vi "总磷总氮通讯.vi"() -> ()   [LabVIEW 2016, in "斯坦道仪器.lvlib"]
uses:
  <vilib>/Utility/config.llb/Write Key (Boolean).vi
  <vilib>/Utility/config.llb/Write Key (String).vi
  <vilib>/Utility/config.llb/Read Key (Boolean).vi
  <vilib>/Utility/config.llb/Read Key (String).vi
  <vilib>/Plasmionique/MB Master/MB_Master/MB_Master.lvclass
  <vilib>/Utility/config.llb/NI_LVConfig.lvlib
  <vilib>/Plasmionique/MB Master/MB Master.lvlib
  <vilib>/ptbypt/NI_PtbyPt.lvlib
panel:
  out "序列号":string
  out "状态告警区":T1
  out "测量数据区":T2 {"单位" items=["ug/L", "mg/L", "ppm", "mg/m3", "cm", "ppb", "ug/m3", "%", "nmol/mol", "umol/mol", "MPN/L", "MPN/100ml", "ng/m3", "NTU", "无量纲", "ms/cm", "us/cm", "℃", "mV", "万个/L"]}
  out "status":bool
  out "关键参数区":T3
  in  "读关键参数区":bool
  in  "读状态告警区":bool
  in  "读测量数据区":bool
  in  "站号":u16(ring) items=["总磷"=1, "氨氮"=3]
  in  "停止":bool
  in  "启动":bool
  in  "控制命令":u16(ring) items=["启动测量"=1, "标样核查"=2, "零点核查"=3, "跨度核查"=4, "空白测试"=5, "平行样测试"=6, "加标回收"=7, "空白校准"=8, "标样校准"=9, "初始化（清洗）"=10, "停止测试"=11, "仪器重启"=12, "校时"=13, "模式设置"=14, "测量间隔设置"=15]
  in  "控制命令参数":u16[](array[numeric]) format="%04xH"
  in  "VISA Resource":refnum<visa-resource-name>
  in  "启用模块":bool
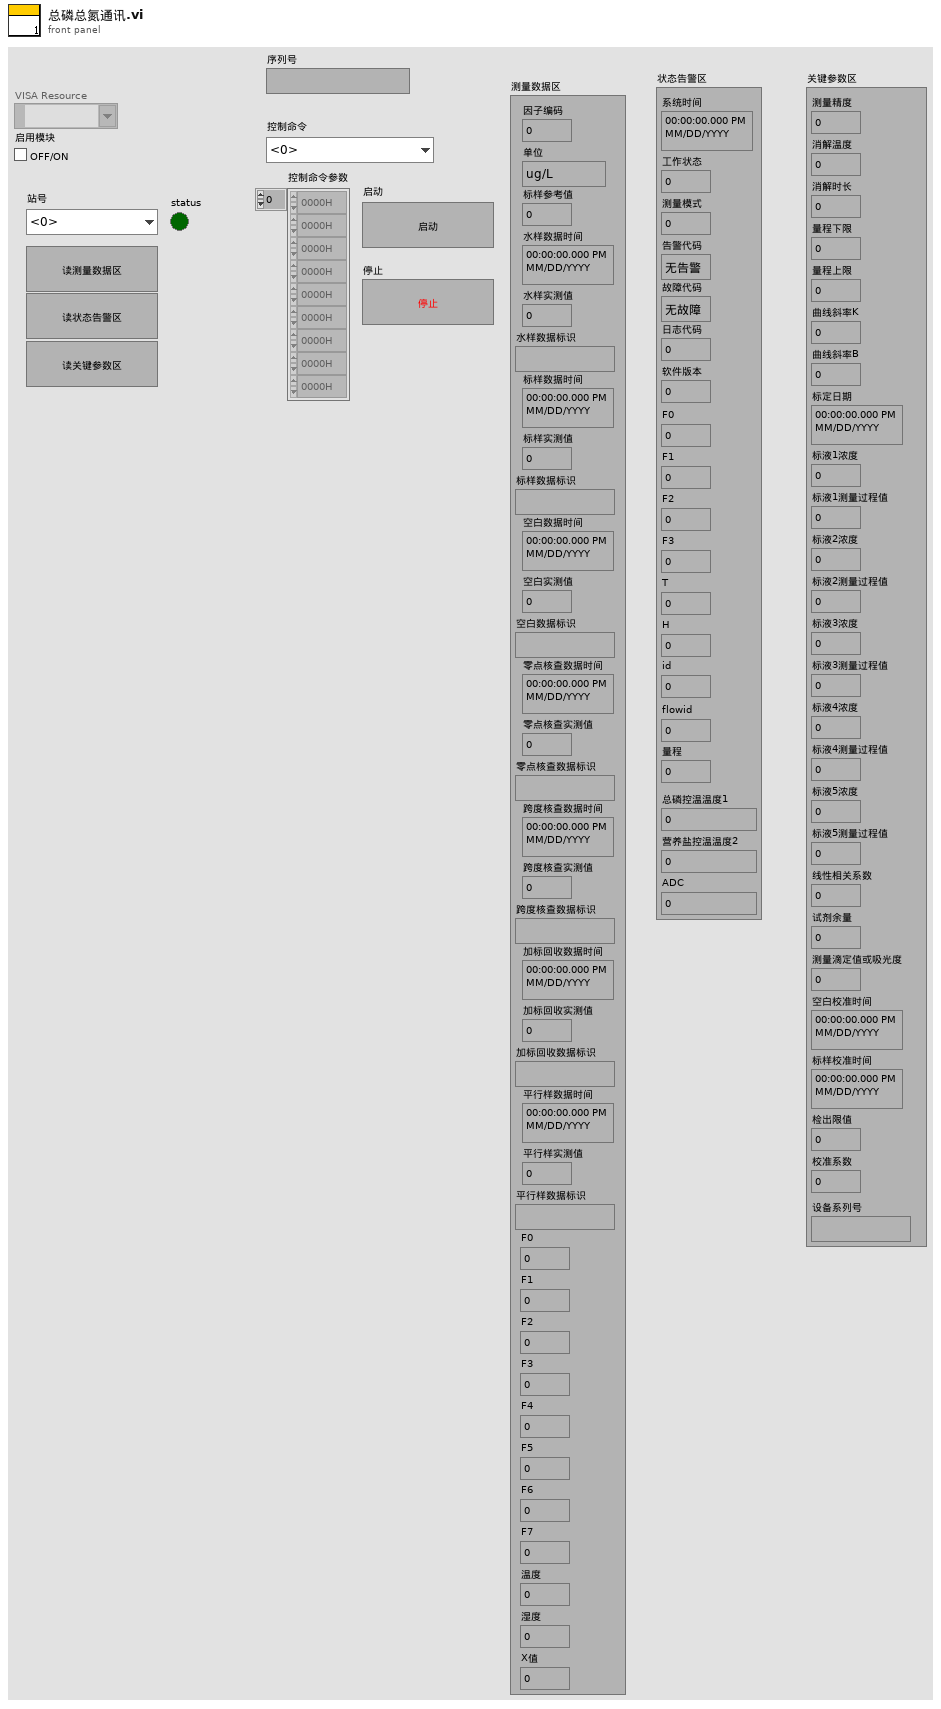
[diagram p1: front panel]
types:
  T1 = cluster{"系统时间":timestamp, "工作状态":u16, "测量模式":u16, "告警代码":enum16{"无告警", "缺试剂告警", "缺水样告警", "缺蒸馏水告警", "缺标液告警", "仪表漏液告警", "标定异常告警", "超量程告警", "加热异常", "低试剂预警", "超上限告警", "超下限告警", "仪表内部其他异常", "滴定异常告警", "电极异常告警", "量程切换告警", "参数设置告警", "PH电极电位异常", "电导率电极异常", "浊度光度异常", "溶解氧电极异常", "溶解氧光强异常", "温度异常告警", "PH异常告警", "溶解氧异常告警", "电导率异常告警", "浊度异常告警", "叶绿素异常告警", "藻密度异常告警", "蓝绿藻异常告警", "ORP异常告警", "氨氮异常告警", "清洁刷异常告警", "SD卡异常告警", "蓝牙异常告警", "Wifi异常告警", "流程异常告警"}, "故障代码":enum16{"无故障", "电机故障", "温度故障", "通讯故障", "滴定故障"}, "日志代码":u16, "软件版本":u16, "F0":sgl, "F1":sgl, "F2":sgl, "F3":sgl, "T":sgl, "H":sgl, "id":u16, "flowid":u16, "量程":u16, "总磷控温温度1":sgl, "营养盐控温温度2":sgl, "ADC":sgl}
  T2 = cluster{"因子编码":u32, "单位":u16, "标样参考值":sgl, "水样数据时间":timestamp, "水样实测值":sgl, "水样数据标识":string, "标样数据时间":timestamp, "标样实测值":sgl, "标样数据标识":string, "空白数据时间":timestamp, "空白实测值":sgl, "空白数据标识":string, "零点核查数据时间":timestamp, "零点核查实测值":sgl, "零点核查数据标识":string, "跨度核查数据时间":timestamp, "跨度核查实测值":sgl, "跨度核查数据标识":string, "加标回收数据时间":timestamp, "加标回收实测值":sgl, "加标回收数据标识":string, "平行样数据时间":timestamp, "平行样实测值":sgl, "平行样数据标识":string, "F0":sgl, "F1":sgl, "F2":sgl, "F3":sgl, "F4":sgl, "F5":sgl, "F6":sgl, "F7":sgl, "温度":sgl, "湿度":sgl, "X值":sgl}
  T3 = cluster{"测量精度":u16, "消解温度":u16, "消解时长":u16, "量程下限":sgl, "量程上限":sgl, "曲线斜率K":sgl, "曲线斜率B":sgl, "标定日期":timestamp, "标液1浓度":sgl, "标液1测量过程值":sgl, "标液2浓度":sgl, "标液2测量过程值":sgl, "标液3浓度":sgl, "标液3测量过程值":sgl, "标液4浓度":sgl, "标液4测量过程值":sgl, "标液5浓度":sgl, "标液5测量过程值":sgl, "线性相关系数":sgl, "试剂余量":u32, "测量滴定值或吸光度":sgl, "空白校准时间":timestamp, "标样校准时间":timestamp, "检出限值":sgl, "校准系数":sgl, "设备系列号":string}
  T4 = typedef "NI_LVConfig.lvlib/Config Data RefNum.ctl" = refnum<k1>
  T5 = enum8{"Enabled", "Disabled", "Disabled and Grayed Out"}
  T6 = cluster{"系统时间":timestamp, "工作状态":enum16{"空闲", "水样测试", "标样核查", "零点核查", "跨度核查", "空白测试", "平行样测试", "加标回收", "空白校准", "标样校准", "初始化（清洗）"}, "测量模式":enum16{"待机", "连续模式", "周期模式", "定点模式", "受控模式", "手动模式"}, "告警代码":enum16{"无告警", "缺试剂告警", "缺水样告警", "缺蒸馏水告警", "缺标液告警", "仪表漏液告警", "标定异常告警", "超量程告警", "加热异常", "低试剂预警", "超上限告警", "超下限告警", "仪表内部其他异常", "滴定异常告警", "电极异常告警", "量程切换告警", "参数设置告警", "PH电极电位异常", "电导率电极异常", "浊度光度异常", "溶解氧电极异常", "溶解氧光强异常", "温度异常告警", "PH异常告警", "溶解氧异常告警", "电导率异常告警", "浊度异常告警", "叶绿素异常告警", "藻密度异常告警", "蓝绿藻异常告警", "ORP异常告警", "氨氮异常告警", "清洁刷异常告警", "SD卡异常告警", "蓝牙异常告警", "Wifi异常告警", "流程异常告警"}, "故障代码":enum16{"无故障", "电机故障", "温度故障", "通讯故障", "滴定故障"}, "日志代码":u16, "软件版本":u16, "F0":sgl, "F1":sgl, "F2":sgl, "F3":sgl, "T":sgl, "H":sgl, "id":u16, "flowid":u16, "量程":u16, "总磷控温温度1":sgl, "营养盐控温温度2":sgl, "ADC":sgl}
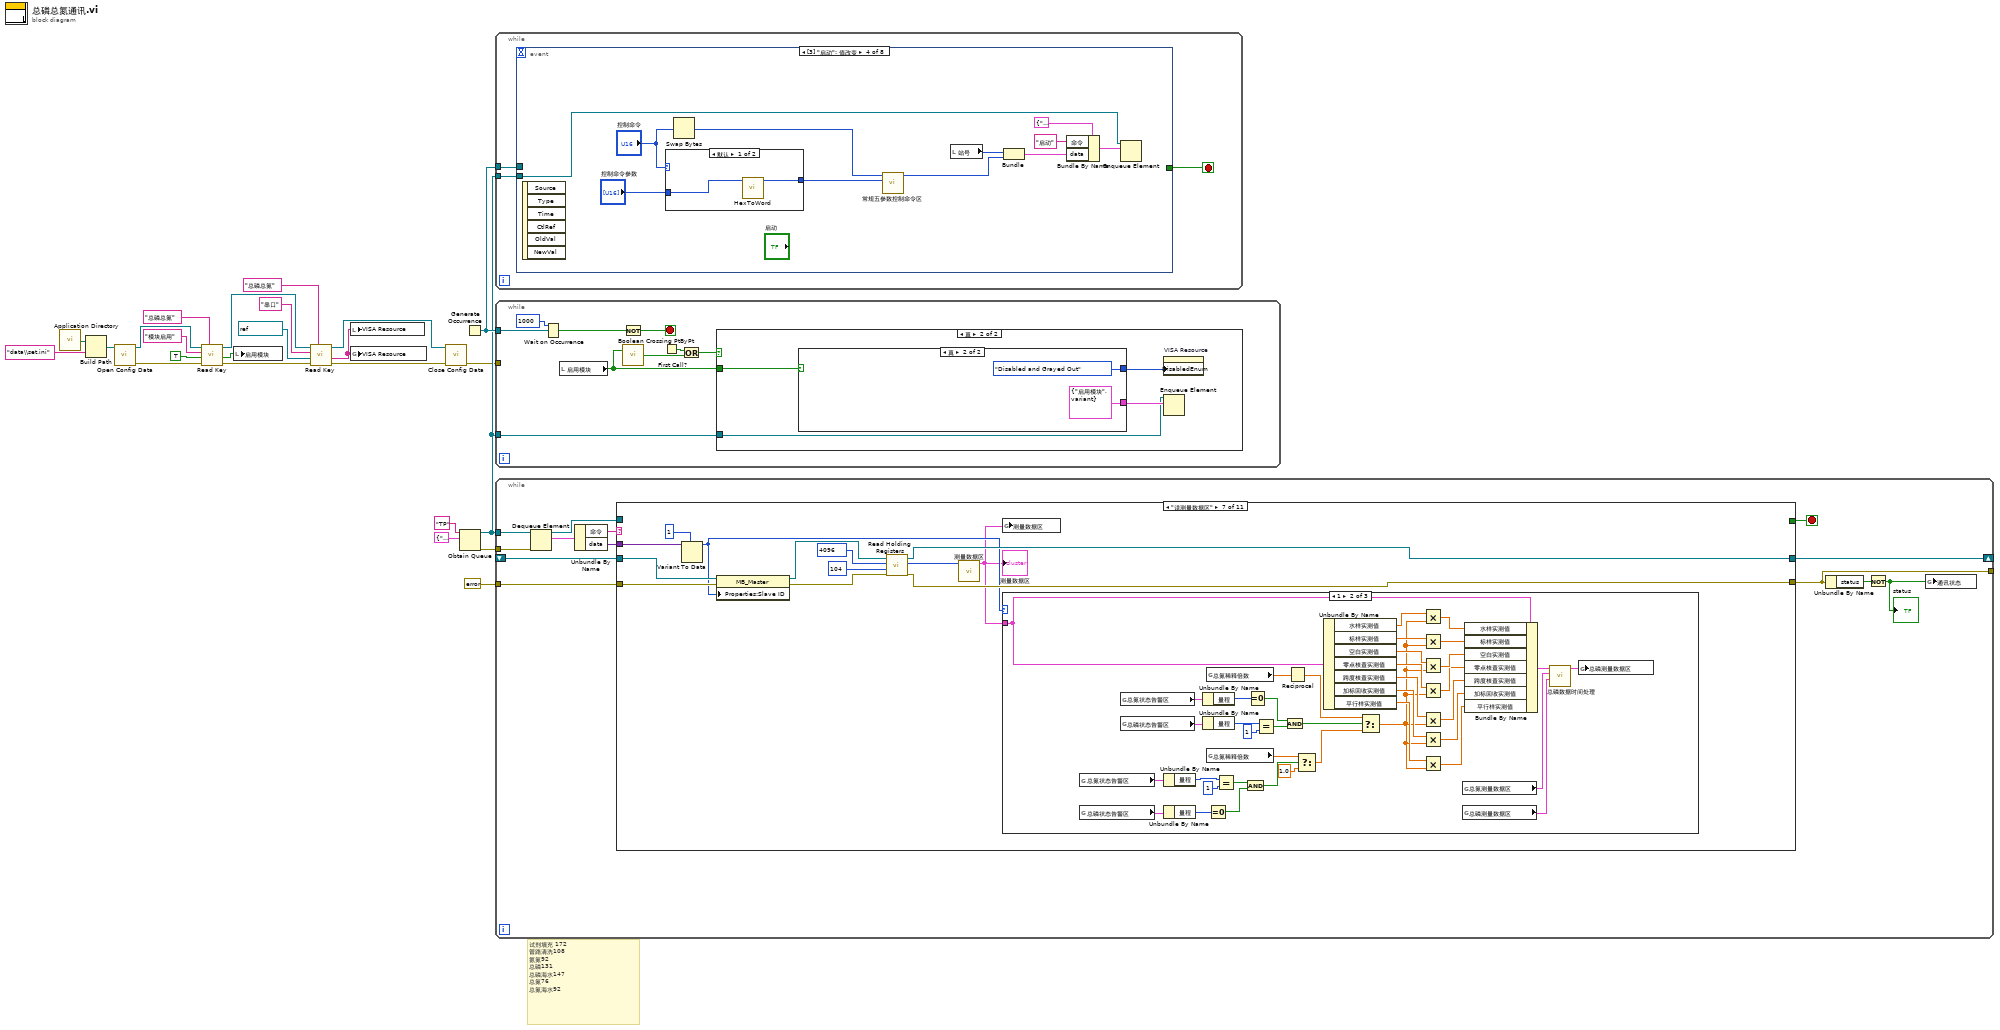
[diagram p0: block diagram]
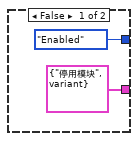
[diagram p3: hidden frame]
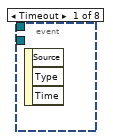
[diagram p4: hidden frame]
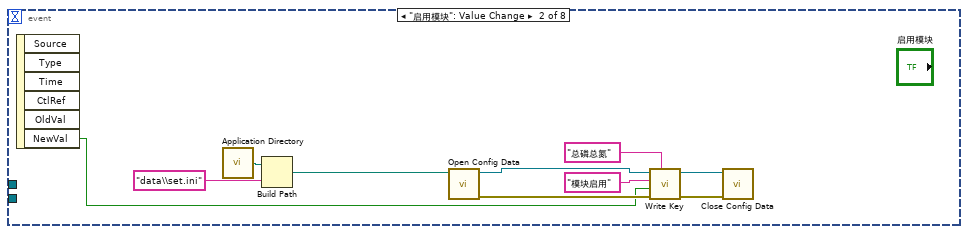
[diagram p5: hidden frame]
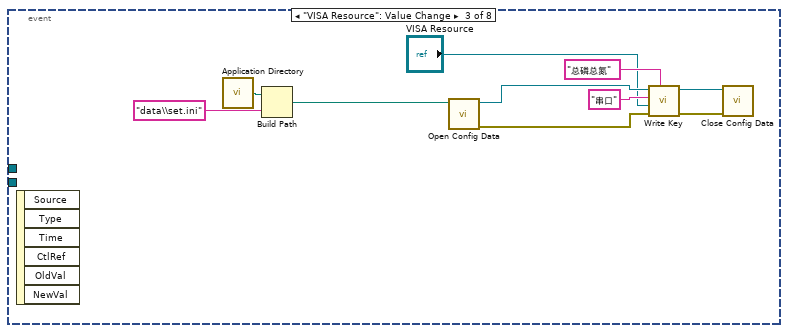
[diagram p6: hidden frame]
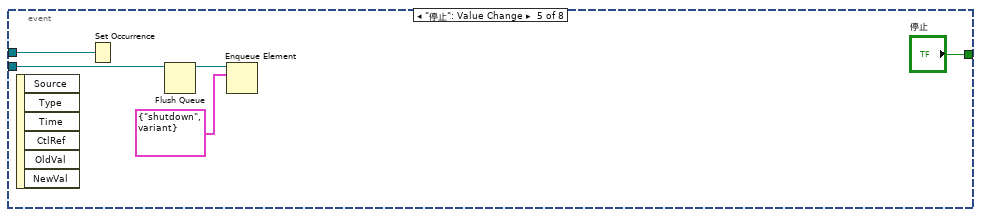
[diagram p8: hidden frame]
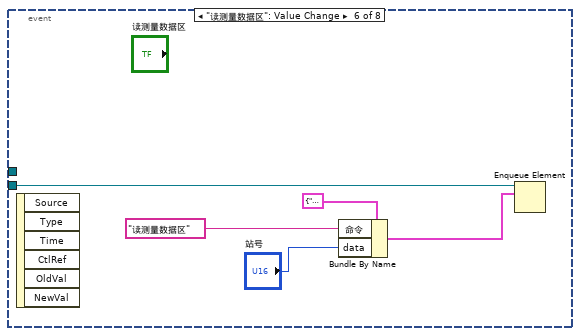
[diagram p9: hidden frame]
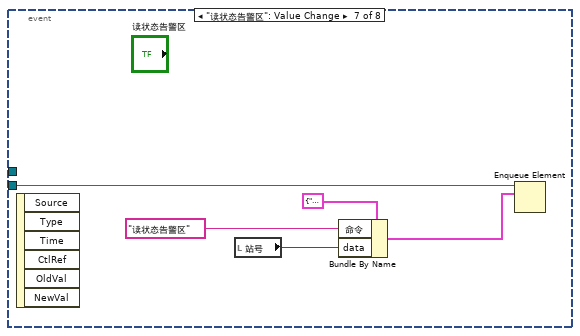
[diagram p10: hidden frame]
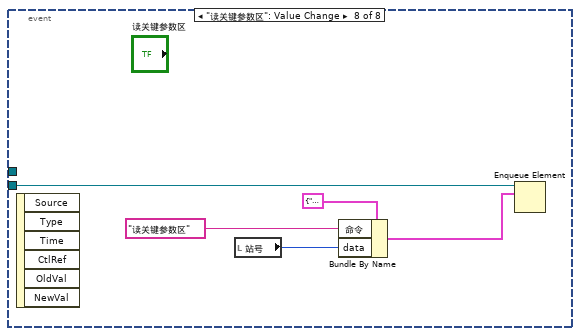
[diagram p11: hidden frame]
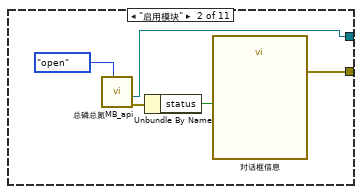
[diagram p13: hidden frame]
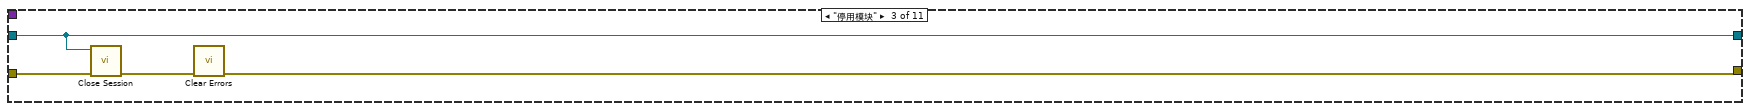
[diagram p14: hidden frame]
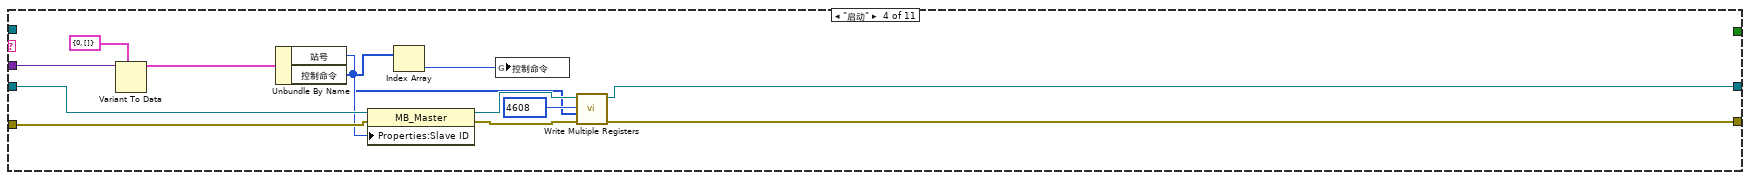
[diagram p15: hidden frame]
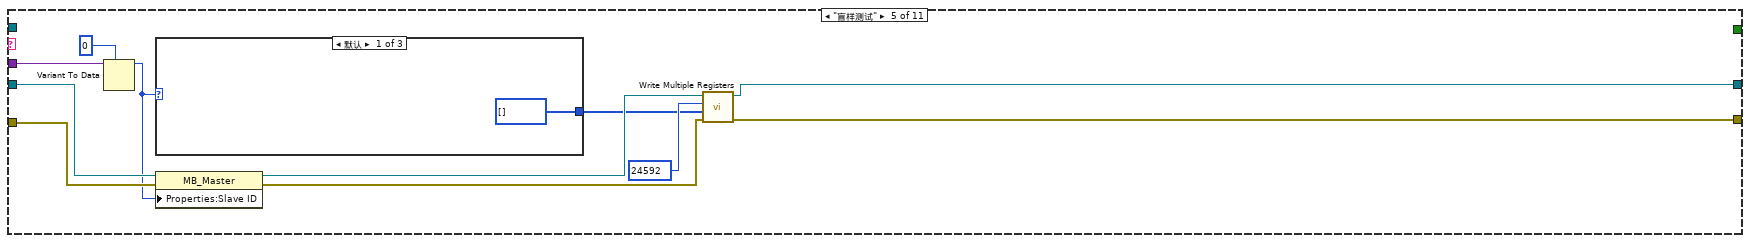
[diagram p16: hidden frame]
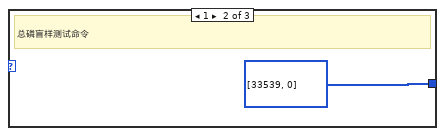
[diagram p17: hidden frame]
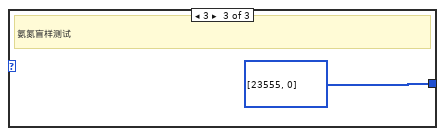
[diagram p18: hidden frame]
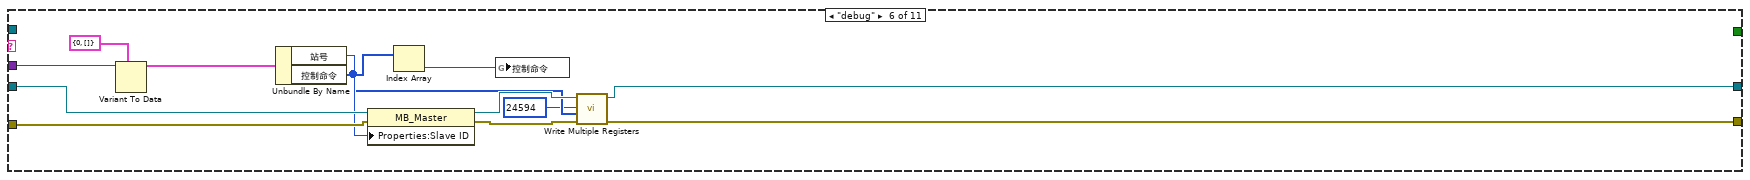
[diagram p19: hidden frame]
diagram:
  # "试剂填充 172 \n管路清洗108\n氨氮92\n总磷131\n总磷海水147\n总氮76\n总氮海水92"
  n1 = call <vilib>:"Application Directory.vi"() -> ("Application Directory"=w12:path)
  n2 = Build Path(base path=w12, name or relative path="data\\set.ini" ("名称或相对路径")) -> (appended path=w13:path)
  n3 = call <vilib>:"Open Config Data.vi"("configuration file path"=w13) -> ("error out"=w18:errorcluster, "refnum"=w17:T4)  [unwired: 8 in, 1 out]
  n4 = call-poly <vilib>:"Read Key.vi"("section"="总磷总氮", "error in (no error)"=w18, "default value"=TRUE ("启用模块"), "key"="模块启用", "refnum"=w17) -> ("error out"=w6:errorcluster, "value"=w9:bool, "refnum out"=w8:T4)  [unwired: 3 in, 1 out]
  n5 = local write "启用模块"(w9) -> ()
  n6 = call-poly <vilib>:"Read Key.vi"("section"="总磷总氮", "error in (no error)"=w6, "default value"=refnum<visa-resource-name> "COM5" ("VISA Resource"), "key"="串口", "refnum"=w8) -> ("error out"=w5:errorcluster, "value"=w1:string, "refnum out"=w7:T4)  [unwired: 3 in, 1 out]
  n7 = local write "VISA Resource"(w1) -> ()
  n8 = global write "VAR总磷总氮全局变量.vi" "VISA Resource"(w1) -> ()
  n9 = call <vilib>:"Close Config Data.vi"("error in (no error)"=w5, "refnum"=w7) -> ("error out"=w10:errorcluster)  [unwired: 8 in, 1 out]
  n10 = Obtain Queue(name (unnamed)="TP" ("名称（未命名）"), element data type=cluster{"命令":string, "data":variant} {"命令"="", "data"=variant}) -> (queue out=w19:refnum<queue>, error out=w22:errorcluster)  [unwired: 3 in, 1 out]
  n11 = Generate Occurrence() -> (w20:refnum<k4>)
  n12 = while {
    tunnel: w19 -> [w27]
    tunnel: w20 -> [w25]
    stop <- w26 stop-if-true
    n13 = event shown="[3] \"启动\": 值改变" {
      selector: _ -> [_ _ _ _ _ _ _ _]
      dyn-events: _ -> [_ _ _ _ _ _ _ _]
      timeout: _ -> [_ _ _ _ _ _ _ _]
      tunnel: w27 -> [_ _ _ w58 w65 w71 w76 w81]
      tunnel: [_ _ _ _ "停止" _ _ _] -> w26
      tunnel: w25 -> [_ _ _ _ w62 _ _ _]
      event Timeout {
        n14 = event-data() -> ()  [unwired: 1 in, 3 out]
      }
      event "启用模块": Value Change {
        n15 = event-data() -> ("NewVal"=w28:bool)  [unwired: 1 in, 5 out]
        n16 = call <vilib>:"Application Directory.vi"() -> ("Application Directory"=w30:path)
        n17 = Build Path(base path=w30, name or relative path="data\\set.ini" ("名称或相对路径")) -> (appended path=w31:path)
        n18 = call <vilib>:"Open Config Data.vi"("configuration file path"=w31) -> ("error out"=w37:errorcluster, "refnum"=w36:T4)  [unwired: 8 in, 1 out]
        n19 = call-poly <vilib>:"Write Key.vi"("section"="总磷总氮", "error in (no error)"=w37, "value"=w28, "key"="模块启用", "refnum"=w36) -> ("error out"=w33:errorcluster, "refnum out"=w29:T4)  [unwired: 4 in, 1 out]
        n20 = call <vilib>:"Close Config Data.vi"("error in (no error)"=w33, "refnum"=w29) -> ()  [unwired: 8 in, 2 out]
      }
      event "VISA Resource": Value Change {
        n21 = event-data() -> ()  [unwired: 1 in, 6 out]
        n22 = call <vilib>:"Application Directory.vi"() -> ("Application Directory"=w40:path)
        n23 = Build Path(base path=w40, name or relative path="data\\set.ini" ("名称或相对路径")) -> (appended path=w41:path)
        n24 = call <vilib>:"Open Config Data.vi"("configuration file path"=w41) -> ("error out"=w47:errorcluster, "refnum"=w46:T4)  [unwired: 8 in, 1 out]
        n25 = call-poly <vilib>:"Write Key.vi"("section"="总磷总氮", "error in (no error)"=w47, "value"="VISA Resource", "key"="串口", "refnum"=w46) -> ("error out"=w43:errorcluster, "refnum out"=w39:T4)  [unwired: 4 in, 1 out]
        n26 = call <vilib>:"Close Config Data.vi"("error in (no error)"=w43, "refnum"=w39) -> ()  [unwired: 8 in, 2 out]
      }
      event "启动": Value Change {
        n27 = event-data() -> ()  [unwired: 1 in, 6 out]
        n28 = case shown="默认" "控制命令" {
          tunnel: "控制命令参数" -> [w60 w61]
          tunnel: [w59 w61] -> w48
          frame Default {
            n29 = call "HexToWord.vi"("数组"=w60) -> ("WORD"=w59:u16[])  [unwired: 10 in]
          }
          frame 13 {
          }
        }
        n30 = Swap Bytes(anything="控制命令") -> (byte swapped=w51:u16)
        n31 = call "常规五参数控制命令区.vi"("控制命令参数"=w48, "控制命令"=w51) -> ("控制命令输出"=w54:u16[])  [unwired: 9 in]
        n32 = local read "站号"() -> (w53:u16)
        n33 = Bundle("站号"=w53, "控制命令输出"=w54) -> (w52:cluster{"站号":u16, "控制命令输出":u16[]})  [unwired: 1 in]
        n34 = Bundle By Name(cluster=cluster{"命令":string, "data":variant} {"命令"="", "data"=variant} ("元素"), "命令"="启动", "data"=w52) -> (w56:cluster{"命令":string, "data":variant})
        n35 = Enqueue Element(queue=w58, element=w56) -> ()  [unwired: 2 in, 3 out]
      }
      event "停止": Value Change {
        n36 = event-data() -> ()  [unwired: 1 in, 6 out]
        n37 = Set Occurrence(w62) -> ()
        n38 = Flush Queue(queue=w65) -> (queue out=w64:refnum<queue>)  [unwired: 1 in, 2 out]
        n39 = Enqueue Element(queue=w64, element=cluster{"命令":string, "data":variant} {"命令"="shutdown", "data"=variant} ("元素")) -> ()  [unwired: 2 in, 3 out]
      }
      event "读测量数据区": Value Change {
        n40 = event-data() -> ()  [unwired: 1 in, 6 out]
        n41 = Bundle By Name(cluster=cluster{"命令":string, "data":variant} {"命令"="", "data"=variant} ("元素"), "命令"="读测量数据区", "data"="站号") -> (w69:cluster{"命令":string, "data":variant})
        n42 = Enqueue Element(queue=w71, element=w69) -> ()  [unwired: 2 in, 3 out]
      }
      event "读状态告警区": Value Change {
        n43 = event-data() -> ()  [unwired: 1 in, 6 out]
        n44 = local read "站号"() -> (w72:u16)
        n45 = Bundle By Name(cluster=cluster{"命令":string, "data":variant} {"命令"="", "data"=variant} ("元素"), "命令"="读状态告警区", "data"=w72) -> (w74:cluster{"命令":string, "data":variant})
        n46 = Enqueue Element(queue=w76, element=w74) -> ()  [unwired: 2 in, 3 out]
      }
      event "读关键参数区": Value Change {
        n47 = event-data() -> ()  [unwired: 1 in, 6 out]
        n48 = local read "站号"() -> (w77:u16)
        n49 = Bundle By Name(cluster=cluster{"命令":string, "data":variant} {"命令"="", "data"=variant} ("元素"), "命令"="读关键参数区", "data"=w77) -> (w79:cluster{"命令":string, "data":variant})
        n50 = Enqueue Element(queue=w81, element=w79) -> ()  [unwired: 2 in, 3 out]
      }
    }
  }
  n51 = while {
    tunnel: w20 -> [w90]
    tunnel: w19 -> [w85]
    tunnel: w10 -> [_]
    stop <- w87 stop-if-true
    n52 = Wait on Occurrence(2:w90, 3:1000 ("毫秒超时(-1)")) -> (0:w88:bool)  [unwired: 1 in]
    n53 = local read "启用模块"() -> (w86:bool)
    n54 = Not(x=w88) -> (.not. x?=w87:bool)
    n55 = call <vilib>:"Boolean Crossing PtByPt.vi"("input"=w86) -> ("crossing"=w83:bool)  [unwired: 2 in]
    n56 = First Call?() -> (First Call?: T/F=w84:bool)
    n57 = Or(x=w84, y=w83) -> (x .or. y?=w82:bool)
    n58 = case shown="真" w82 {
      tunnel: w86 -> [_ w93]
      tunnel: w85 -> [_ w92]
      frame False {
      }
      frame True {
        n59 = case shown="真" w93 {
          tunnel: [cluster{"命令":string, "data":variant} {"命令"="停用模块", "data"=variant} ("元素") cluster{"命令":string, "data":variant} {"命令"="启用模块", "data"=variant} ("元素")] -> w94
          tunnel: [T5."Enabled" ("禁用") T5."Disabled and Grayed Out" ("禁用")] -> w91
          frame False {
          }
          frame True {
          }
        }
        n60 = property on="VISA Resource" class="VISAName"("DisabledEnum"=w91) -> ()  [unwired: 2 in, 2 out]
        n61 = Enqueue Element(queue=w92, element=w94) -> ()  [unwired: 2 in, 3 out]
      }
    }
  }
  n62 = while {
    tunnel: w19 -> [w111]
    tunnel: w22 -> [w110]
    shift-right: [w108] -> _
    shift-left: _ -> [w107]
    tunnel: errorcluster {"status"=FALSE, "code"=0, "source"=""} ("error out") -> [w106]
    tunnel: [w101] -> _
    stop <- w109 stop-if-true
    n63 = Dequeue Element(queue=w111, error in (no error)=w110) -> (queue out=w102:refnum<queue>, element=w104:cluster{"命令":string, "data":variant})  [unwired: 1 in, 2 out]
    n64 = Unbundle By Name(w104) -> ("命令"=w105:string, "data"=w103:variant)
    n65 = case shown="\"读测量数据区\"" w105 {
      tunnel: w103 -> [_ _ _ w132 w143 w160 w170 w222 w238 w252 _]
      tunnel: w102 -> [_ _ _ _ _ _ _ _ _ _ w265]
      tunnel: [_ _ _ _ _ _ _ _ _ _ TRUE] -> w109
      tunnel: [w112 w114 w119 w135 w146 w162 w174 w231 w245 w259 w261] -> w108
      tunnel: [w113 w117 w120 w134 w145 w161 w175 w220 w246 w260 w262] -> w101
      tunnel: w107 -> [w112 _ w119 w131 w142 w159 w169 w225 w241 w255 w261]
      tunnel: w106 -> [w113 _ w122 w128 w139 w156 w167 w226 w242 w256 w263]
      frame Default {
      }
      frame "启用模块" {
        n66 = call "总磷总氮MB_api.vi"("STEP"=enum16{"open", "read", "write", "close"}."open") -> ("error out"=w115:errorcluster, "MB session out"=w114:refnum<class "MB_Master.lvclass">)  [unwired: 7 in, 2 out]
        n67 = Unbundle By Name(w115) -> ("status"=w118:bool)
        n68 = call "对话框信息"("Enable"=w118) -> ("error out"=w117:errorcluster)  [unwired: 9 in, 1 out]
      }
      frame "停用模块" {
        n69 = call-dynamic "Close Session.vi"("error in (no error)"=w122, "MB session in"=w119) -> ("error out"=w121:errorcluster)  [unwired: 9 in]
        n70 = call <vilib>:"Clear Errors.vi"("error in (no error)"=w121) -> ("error out"=w120:errorcluster)  [unwired: 5 in, 1 out]
      }
      frame "启动" {
        n71 = Variant To Data(type=cluster{"站号":u16, "控制命令":u16[]} {"站号"=0, "控制命令"=[]} ("输出簇"), Variant=w132) -> (data=w126:cluster{"站号":u16, "控制命令":u16[]})  [unwired: 1 in, 1 out]
        n72 = Unbundle By Name(w126) -> ("站号"=w125:u16, "控制命令"=w123:u16[])
        n73 = property class="MB_Master"(reference=w131, error in=w128, "Properties:Slave ID"=w125) -> (reference out=w130:refnum<class "MB_Master.lvclass">, error out=w129:errorcluster)
        n74 = Index Array(array=w123) -> (element=w124:u16)  [unwired: 1 in]
        n75 = global write "VAR总磷总氮全局变量.vi" "控制命令"(w124) -> ()
        n76 = call <vilib>:"Write Multiple Registers.vi"("error in (no error)"=w129, "values"=w123, "starting address"=u16 4608, "MB session in"=w130) -> ("error out"=w134:errorcluster, "MB session out"=w135:refnum<class "MB_Master.lvclass">)  [unwired: 6 in]
      }
      frame "盲样测试" {
        n77 = Variant To Data(type=0, Variant=w143) -> (data=w136:i32)  [unwired: 1 in, 1 out]
        n78 = case shown="默认" w136 {
          tunnel: [u16[] [] ("values") u16[] [33539, 0] ("values") u16[] [23555, 0] ("values")] -> w138
          frame Default {
          }
          frame 1 {
            # "总磷盲样测试命令"
          }
          frame 3 {
            # "氨氮盲样测试"
          }
        }
        n79 = property class="MB_Master"(reference=w142, error in=w139, "Properties:Slave ID"=w136) -> (reference out=w141:refnum<class "MB_Master.lvclass">, error out=w140:errorcluster)
        n80 = call <vilib>:"Write Multiple Registers.vi"("error in (no error)"=w140, "values"=w138, "starting address"=u16 24592, "MB session in"=w141) -> ("error out"=w145:errorcluster, "MB session out"=w146:refnum<class "MB_Master.lvclass">)  [unwired: 6 in]
      }
      frame "debug" {
        n81 = Variant To Data(type=cluster{"站号":u16, "控制命令":u16[]} {"站号"=0, "控制命令"=[]} ("输出簇"), Variant=w160) -> (data=w154:cluster{"站号":u16, "控制命令":u16[]})  [unwired: 1 in, 1 out]
        n82 = Unbundle By Name(w154) -> ("站号"=w153:u16, "控制命令"=w151:u16[])
        n83 = property class="MB_Master"(reference=w159, error in=w156, "Properties:Slave ID"=w153) -> (reference out=w158:refnum<class "MB_Master.lvclass">, error out=w157:errorcluster)
        n84 = Index Array(array=w151) -> (element=w152:u16)  [unwired: 1 in]
        n85 = global write "VAR总磷总氮全局变量.vi" "控制命令"(w152) -> ()
        n86 = call <vilib>:"Write Multiple Registers.vi"("error in (no error)"=w157, "values"=w151, "starting address"=u16 24594, "MB session in"=w158) -> ("error out"=w161:errorcluster, "MB session out"=w162:refnum<class "MB_Master.lvclass">)  [unwired: 6 in]
      }
      frame "读测量数据区" {
        n87 = Variant To Data(type=u8 1 ("Slave ID"), Variant=w170) -> (data=w164:u8)  [unwired: 1 in, 1 out]
        n88 = property class="MB_Master"(reference=w169, error in=w167, "Properties:Slave ID"=w164) -> (reference out=w168:refnum<class "MB_Master.lvclass">, error out=w166:errorcluster)
        n89 = call <vilib>:"Read Holding Registers.vi"("error in (no error)"=w166, "quantity"=u16 104, "starting address"=u16 4096, "MB session in"=w168) -> ("error out"=w175:errorcluster, "Registers"=w165:u16[], "MB session out"=w174:refnum<class "MB_Master.lvclass">)  [unwired: 5 in]
        n90 = call "测量数据区.vi"("数组"=w165) -> ("测量数据区"=w163:T2)  [unwired: 10 in]
        "测量数据区" <- w163
        n91 = global write "VAR总磷总氮全局变量.vi" "测量数据区"(w163) -> ()
        n92 = case shown="1" w164 {
          tunnel: w163 -> [_ w216 w217]
          frame 0, Default {
          }
          frame 1 {
            n93 = global read "VAR总磷总氮全局变量.vi" "总氮状态告警区"() -> (w183:T6)
            n94 = global read "VAR总磷总氮全局变量.vi" "总磷状态告警区"() -> (w184:T6)
            n95 = global read "VAR总磷总氮全局变量.vi" "总氮状态告警区"() -> (w195:T6)
            n96 = global read "VAR总磷总氮全局变量.vi" "总磷状态告警区"() -> (w194:T6)
            n97 = Unbundle By Name(w183) -> ("量程"=w182:u16)
            n98 = Unbundle By Name(w184) -> ("量程"=w180:u16)
            n99 = Unbundle By Name(w195) -> ("量程"=w193:u16)
            n100 = Unbundle By Name(w194) -> ("量程"=w192:u16)
            n101 = global read "VAR总磷总氮全局变量.vi" "总氮稀释倍数"() -> (w201:dbl)
            n102 = global read "VAR总磷总氮全局变量.vi" "总氮稀释倍数"() -> (w178:dbl)
            n103 = Equal To 0?(x=w180) -> (x = 0?=w185:bool)
            n104 = Equal?(x=w182, y=u16 1) -> (x = y?=w186:bool)
            n105 = And(x=w186, y=w185) -> (x .and. y?=w179:bool)
            n106 = Equal To 0?(x=w193) -> (x = 0?=w189:bool)
            n107 = Equal?(x=w192, y=u16 1) -> (x = y?=w190:bool)
            n108 = And(x=w189, y=w190) -> (x .and. y?=w188:bool)
            n109 = Reciprocal(x=w201) -> (1/x=w187:dbl)
            n110 = Select(t=w178, s=w179, f=1.0) -> (s? t:f=w176:dbl)
            n111 = Unbundle By Name(w216) -> ("水样实测值"=w215:sgl, "标样实测值"=w213:sgl, "空白实测值"=w211:sgl, "零点核查实测值"=w209:sgl, "跨度核查实测值"=w207:sgl, "加标回收实测值"=w205:sgl, "平行样实测值"=w203:sgl)
            n112 = Select(t=w187, s=w188, f=w176) -> (s? t:f=w200:dbl)
            n113 = Multiply(x=w215, y=w200) -> (x*y=w214:dbl)
            n114 = Multiply(x=w213, y=w200) -> (x*y=w212:dbl)
            n115 = Multiply(x=w211, y=w200) -> (x*y=w210:dbl)
            n116 = Multiply(x=w209, y=w200) -> (x*y=w208:dbl)
            n117 = Multiply(x=w207, y=w200) -> (x*y=w206:dbl)
            n118 = Multiply(x=w205, y=w200) -> (x*y=w204:dbl)
            n119 = Multiply(x=w203, y=w200) -> (x*y=w202:dbl)
            n120 = global read "VAR总磷总氮全局变量.vi" "总氮测量数据区"() -> (w198:T2)
            n121 = global read "VAR总磷总氮全局变量.vi" "总磷测量数据区"() -> (w196:T2)
            n122 = Bundle By Name(cluster=w216, "水样实测值"=w214, "标样实测值"=w212, "空白实测值"=w210, "零点核查实测值"=w208, "跨度核查实测值"=w206, "加标回收实测值"=w204, "平行样实测值"=w202) -> (w199:T2)
            n123 = call "总磷数据时间处理.vi"("总磷修正数据输入"=w196, "总氮原始数据"=w198, "总磷原始数据"=w199) -> ("总磷修正数据输出"=w197:T2)  [unwired: 8 in]
            n124 = global write "VAR总磷总氮全局变量.vi" "总磷测量数据区"(w197) -> ()
          }
          frame 2 {
            n125 = global write "VAR总磷总氮全局变量.vi" "总氮测量数据区"(w217) -> ()
          }
        }
      }
      frame "读状态告警区" {
        n126 = Variant To Data(type=u8 1 ("Slave ID"), Variant=w222) -> (data=w227:u8)  [unwired: 1 in, 1 out]
        n127 = property class="MB_Master"(reference=w225, error in=w226, "Properties:Slave ID"=w227) -> (reference out=w224:refnum<class "MB_Master.lvclass">, error out=w223:errorcluster)
        n128 = call <vilib>:"Read Holding Registers.vi"("error in (no error)"=w223, "quantity"=u16 29, "starting address"=u16 4224, "MB session in"=w224) -> ("error out"=w220:errorcluster, "Registers"=w221:u16[], "MB session out"=w231:refnum<class "MB_Master.lvclass">)  [unwired: 5 in]
        n129 = call "状态告警区.vi"("数组"=w221) -> ("状态告警区"=w218:T6)  [unwired: 10 in]
        "状态告警区" <- w218
        n130 = Unbundle By Name(w218) -> ("id"=w219:u16)
        n131 = global write "VAR总磷总氮全局变量.vi" "状态告警区"(w218) -> ()
        n132 = case shown="76" w219 {
          tunnel: w218 -> [_ w232 w233]
          frame 0, Default {
          }
          frame 131 {
            n133 = global write "VAR总磷总氮全局变量.vi" "总磷状态告警区"(w232) -> ()
          }
          frame 76 {
            n134 = global write "VAR总磷总氮全局变量.vi" "总氮状态告警区"(w233) -> ()
          }
        }
      }
      frame "读关键参数区" {
        n135 = Variant To Data(type=u8 1 ("Slave ID"), Variant=w238) -> (data=w236:u8)  [unwired: 1 in, 1 out]
        n136 = property class="MB_Master"(reference=w241, error in=w242, "Properties:Slave ID"=w236) -> (reference out=w240:refnum<class "MB_Master.lvclass">, error out=w239:errorcluster)
        n137 = call <vilib>:"Read Holding Registers.vi"("error in (no error)"=w239, "quantity"=u16 19, "starting address"=u16 4256, "MB session in"=w240) -> ("error out"=w246:errorcluster, "Registers"=w235:u16[], "MB session out"=w245:refnum<class "MB_Master.lvclass">)  [unwired: 5 in]
        n138 = call "关键参数区.vi"("数组"=w235) -> ("关键参数区"=w234:T3)  [unwired: 10 in]
        "关键参数区" <- w234
        n139 = global write "VAR总磷总氮全局变量.vi" "关键参数区"(w234) -> ()
      }
      frame "读序列号" {
        n140 = Variant To Data(type=u8 1 ("Slave ID"), Variant=w252) -> (data=w250:u8)  [unwired: 1 in, 1 out]
        n141 = property class="MB_Master"(reference=w255, error in=w256, "Properties:Slave ID"=w250) -> (reference out=w254:refnum<class "MB_Master.lvclass">, error out=w253:errorcluster)
        n142 = call <vilib>:"Read Holding Registers.vi"("error in (no error)"=w253, "quantity"=u16 6, "starting address"=u16 3, "MB session in"=w254) -> ("error out"=w260:errorcluster, "Registers"=w249:u16[], "MB session out"=w259:refnum<class "MB_Master.lvclass">)  [unwired: 5 in]
        n143 = call "HexToString.vi"("数组"=w249) -> ("STRING"=w248:string[])  [unwired: 10 in]
        n144 = Index Array(array=w248) -> (element=w247:string)  [unwired: 1 in]
        "序列号" <- w247
        n145 = global write "VAR总磷总氮全局变量.vi" "序列号"(w247) -> ()
      }
      frame "shutdown" {
        n146 = call-dynamic "Close Session.vi"("error in (no error)"=w263, "MB session in"=w261) -> ("error out"=w262:errorcluster)  [unwired: 9 in]
        n147 = Flush Queue(queue=w265) -> (queue out=w264:refnum<queue>)  [unwired: 1 in, 2 out]
        n148 = Release Queue(queue=w264) -> ()  [unwired: 2 in, 3 out]
      }
    }
    n149 = Unbundle By Name(w101) -> ("status"=w100:bool)
    n150 = Not(x=w100) -> (.not. x?=w99:bool)
    "status" <- w99
    n151 = global write "VAR总磷总氮全局变量.vi" "通讯状态"(w99) -> ()
  }
